vi "FlatToRichcif_template_SetNumericRequest.vi"(5 "OutputClusterType":T1, 11 "InputCluster":T2) -> (3 "OutputCluster":T1)   [LabVIEW 2021, in "Template_client.lvlib"]
uses:
  cif_template_SetNumericRequest_Flat.ctl
  cif_template_SetNumericRequest.ctl
  Template_client.lvlib
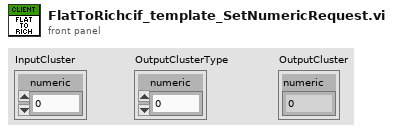
[diagram p1: front panel]
types:
  T1 = typedef "Template_client.lvlib/cif_template_SetNumericRequest.ctl" = cluster{"numeric":i32}
  T2 = typedef "Template_client.lvlib/cif_template_SetNumericRequest_Flat.ctl" = cluster{"numeric":i32}
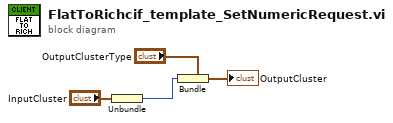
[diagram p0: block diagram]
diagram:
  n1 = Unbundle "Unbundle"("InputCluster") -> ("numeric"=w1:i32)
  n2 = Bundle "Bundle"(cluster="OutputClusterType", "numeric"=w1) -> (→"OutputCluster":T1)
